vi "average tempature.vi"() -> ()   [LabVIEW 2014]
panel:
  out "Waveform Chart":dbl(graph)
  in  "Boolean":bool
  out "Numeric":dbl
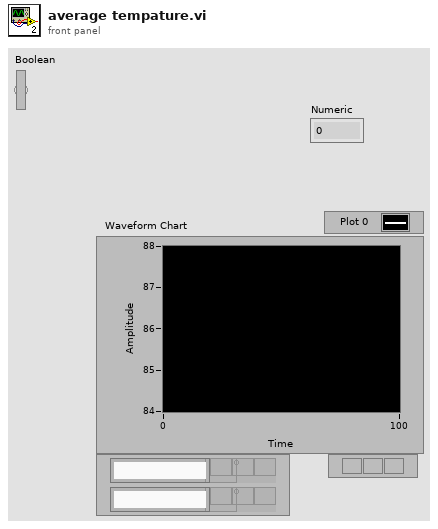
[diagram p1: front panel]
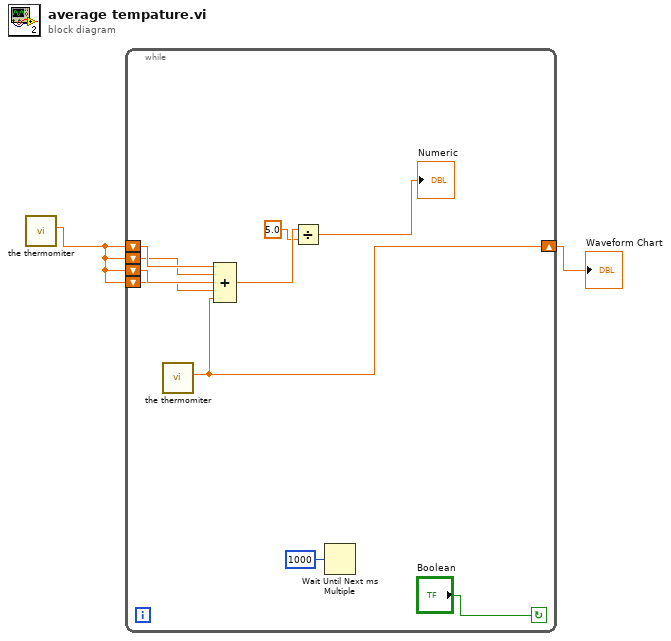
[diagram p0: block diagram]
diagram:
  n1 = call "the thermomiter.vi"() -> ("Temperature"=w2:dbl)  [unwired: 10 in, 1 out]
  n2 = while {
    shift-right: [w6] -> w1
    shift-left: w2 -> [w10]
    shift-left: w2 -> [w9]
    shift-left: w2 -> [w8]
    shift-left: w2 -> [w7]
    stop <- "Boolean" continue-if-true
    n3 = call "the thermomiter.vi"() -> ("Temperature"=w6:dbl)  [unwired: 10 in, 1 out]
    n4 = Compound Arithmetic op=ADD(w10, w9, w8, w7, w6) -> (w5:dbl)
    n5 = Divide(x=w5, y=5.0 ("x")) -> (x/y=→"Numeric":dbl)
    n6 = Wait Until Next ms Multiple(millisecond multiple=u32 1000) -> ()  [unwired: 1 out]
  }
  "Waveform Chart" <- w1
